vi "AVMPanelPan.vi"(8 "error in (no error)":errorcluster caption="entrée d'erreur (pas d'erreur)", 11 "LeafMagnetometer.lvclass":refnum<class "LeafMagnetometer.lvclass">) -> (0 "error out":errorcluster caption="sortie d'erreur", 3 "LeafMagnetometer.lvclass Out":refnum<class "LeafMagnetometer.lvclass">)   [LabVIEW 2012, in "LeafMagnetometer.lvclass"]
uses:
  LeafMagnetometer.lvclass
  LeafMagnetometer.lvclass/LeafMagnetometer.ctl
  BaseDevice/Accessor/GetClassEvent.vi
panel:
  in  "Av Samples":u32=1 caption="Averaged Samples" min=1 max=100000 step=1
  out "Total":dbl format="%.3f"
  in  "Stop":bool
  in  "MiseAJour":bool
  out "Init Program":bool
  # "Twinleaf Magnetometer"
  # "this MUST labeled with class name"
  # "vertical minimum Panel size must be set to desired size"
  # "this MUST be present and labeled \"Stop\""
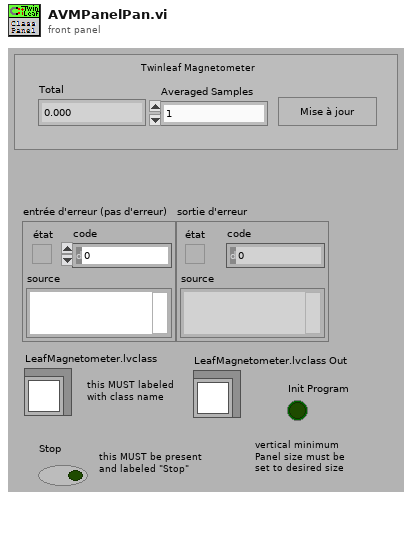
[diagram p1: front panel]
types:
  T1 = cluster{"Name":string, "Waveform":cluster{"start":dbl, "dt":dbl, "Timeseries":dbl[][]}}[][]
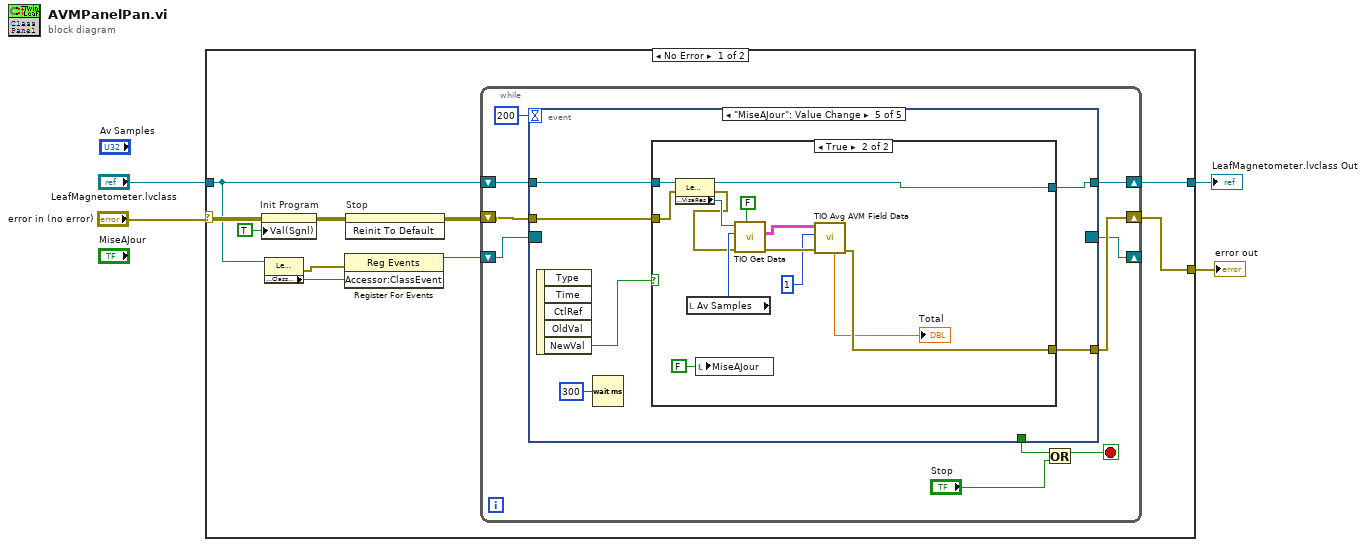
[diagram p0: block diagram]
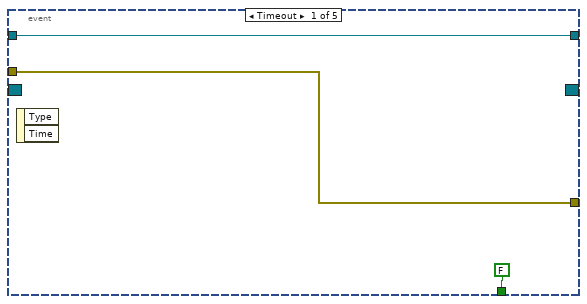
[diagram p2: hidden frame]
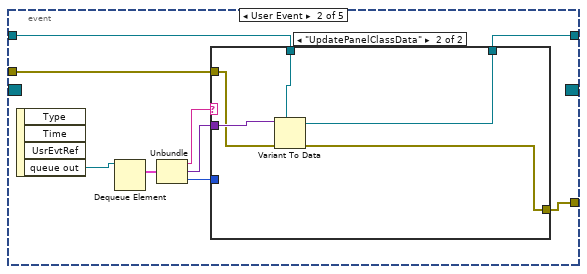
[diagram p3: hidden frame]
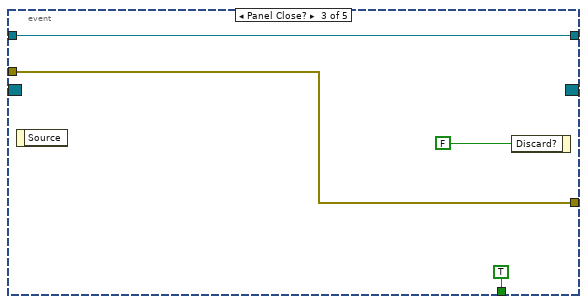
[diagram p5: hidden frame]
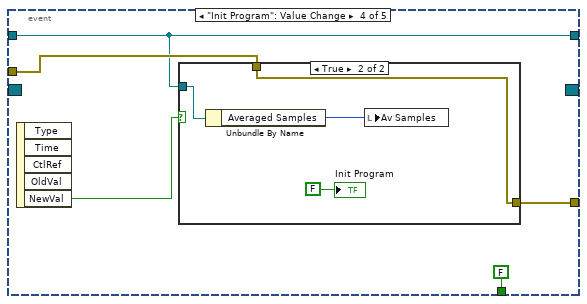
[diagram p6: hidden frame]
diagram:
  n1 = case shown="No Error" "error in (no error)" {
    selector: "error in (no error)" -> [w11 w80]
    tunnel: [w14 w80] -> w3
    tunnel: "LeafMagnetometer.lvclass" -> [w6 w79]
    tunnel: [w12 w79] -> w1
    frame No Error {
      n2 = property on="Init Program" class="Bool (strict)"(error in=w11, "Val(Sgnl)"=TRUE ("Valeur (Signalisation)")) -> (error out=w10:errorcluster)  [unwired: 1 in, 1 out]
      n3 = property class="LeafMagnetometer.lvclass"(reference=w6) -> (error out=w8:errorcluster, "Accessor:ClassEvent"=w7:refnum<user-event>)  [unwired: 1 in, 1 out]
      n4 = register-events(error in=w8, w7) -> (reference out=w5:refnum<event-registration>)  [unwired: 1 in, 1 out]
      n5 = invoke on="Stop" class="Bool (strict)" method="Reinit To Default"(error in=w10) -> (error out=w9:errorcluster)  [unwired: 2 in, 2 out]
      n6 = while {
        shift-right: [w22] -> w14
        shift-left: w9 -> [w23]
        shift-right: [w19] -> w12
        shift-left: w6 -> [w21]
        shift-right: [w15] -> _
        shift-left: w5 -> [w16]
        stop <- w18 stop-if-true
        n7 = event shown="[4] \"MiseAJour\": Value Change" {
          selector: w16 -> [_ _ _ _ _]
          dyn-events: [_ _ _ _ _] -> w15
          timeout: 200 -> [_ _ _ _ _]
          tunnel: w23 -> [w25 w35 w45 w51 w59]
          tunnel: [w25 w29 w45 w50 w58] -> w22
          tunnel: w21 -> [w26 w36 w44 w48 w60]
          tunnel: [FALSE _ TRUE FALSE _] -> w20
          tunnel: [w26 w28 w44 w48 w61] -> w19
          event Timeout {
            n8 = event-data() -> ()  [unwired: 1 in, 2 out]
          }
          event User Event {
            n9 = event-data() -> ("queue out"=w33:refnum<queue>)  [unwired: 1 in, 3 out]
            n10 = Dequeue Element(queue=w33) -> (element=w34:cluster{"Message":string, "Data":variant, i32})  [unwired: 2 in, 3 out]
            n11 = Unbundle(w34) -> ("Message"=w32:string, "Data"=w31:variant, w30:i32)
            n12 = case shown="\"UpdatePanelClassData\"" w32 {
              tunnel: w35 -> [w37 w40]
              tunnel: w31 -> [_ w43]
              tunnel: w36 -> [w38 w42]
              tunnel: [w38 w41] -> w28
              tunnel: [w37 w39] -> w29
              tunnel: w30 -> [_ _]
              frame "Faux", Default {
              }
              frame "UpdatePanelClassData" {
                n13 = Variant To Data(error in=w40, type=w42, Variant=w43) -> (data=w41:refnum<class "LeafMagnetometer.lvclass">, error out=w39:errorcluster)
              }
            }
          }
          event Panel Close? {
            n14 = event-data() -> ()  [unwired: 1 in, 1 out]
            n15 = event-data("Discard?"=FALSE ("Rejeter ?")) -> ()  [unwired: 1 in, 1 out]
          }
          event "Init Program": Value Change {
            n16 = event-data() -> ("NewVal"=w52:bool)  [unwired: 1 in, 4 out]
            n17 = case shown="True" w52 {
              tunnel: w51 -> [w53 w56]
              tunnel: [w53 w56] -> w50
              tunnel: w48 -> [_ w55]
              frame False {
              }
              frame True {
                n18 = Unbundle By Name(w55) -> ("Averaged Samples"=w54:u32)
                n19 = local write "Av Samples"(w54) -> ()
                "Init Program" <- FALSE
              }
            }
          }
          event "MiseAJour": Value Change {
            n20 = event-data() -> ("NewVal"=w62:bool)  [unwired: 1 in, 4 out]
            n21 = Wait (ms)(milliseconds to wait=u32 300 ("attente (ms)")) -> ()  [unwired: 1 out]
            n22 = case shown="True" w62 {
              tunnel: [w65 w76] -> w61
              tunnel: w60 -> [w65 w77]
              tunnel: w59 -> [w64 w70]
              tunnel: [w64 w68] -> w58
              frame False {
              }
              frame True {
                n23 = property class="LeafMagnetometer.lvclass"(reference=w77, error in=w70) -> (reference out=w76:refnum<class "LeafMagnetometer.lvclass">, error out=w69:errorcluster, "Accessor:VisaRes"=w75:refnum<visa-resource-name>)
                n24 = local read "Av Samples"() -> (w71:u32)
                n25 = local write "MiseAJour"(FALSE ("MiseAJour")) -> ()
                n26 = call <userlib>:"TIO Get Data.vi"("Type(T:GMR)"=FALSE, "entrée d'erreur (pas d'erreur)"=w69, "Samples Count"=w71, "Nom de ressource VISA"=w75) -> ("sortie d'erreur"=w74:errorcluster, "Tableau"=w73:T1)  [unwired: 5 in, 1 out]
                n27 = call <userlib>:"TIO Avg AVM Field Data.vi"("entrée d'erreur (pas d'erreur)"=w74, "Component Index"=1, "Tableau"=w73) -> ("sortie d'erreur"=w68:errorcluster, "Total Average"=→"Total":dbl)  [unwired: 5 in, 2 out]
              }
            }
          }
        }
        n28 = Or(x=w20, y="Stop") -> (x .or. y?=w18:bool)
      }
    }
    frame Error {
    }
  }
  "error out" <- w3
  "LeafMagnetometer.lvclass Out" <- w1
